vi "S2C_UNITHERM_Proc_Commands.vi"(7 "VI_Ref":refnum<vi>, 8 "Error In":errorcluster, 10 "Settings":T1, 11 "Q-Ref":refnum<queue>) -> (0 "Error Out":errorcluster, 2 "Stop?":bool, 3 "Response":variant)   [LabVIEW 2024]
uses:
  S2C_UNITHERM_Proc_Globals.vi
  _Shared/S2C_Shared_Proc_Globals.vi
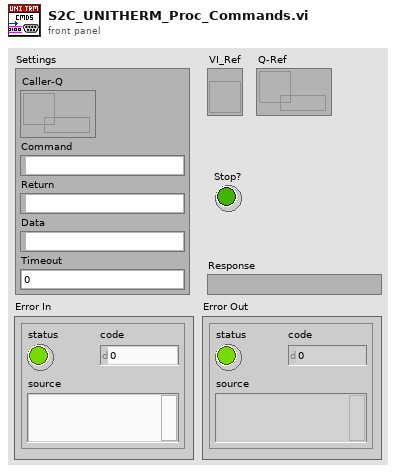
[diagram p1: front panel]
types:
  T1 = cluster{"Caller-Q":refnum<queue>, "Command":string, "Return":string, "Data":variant, "Timeout":dbl}
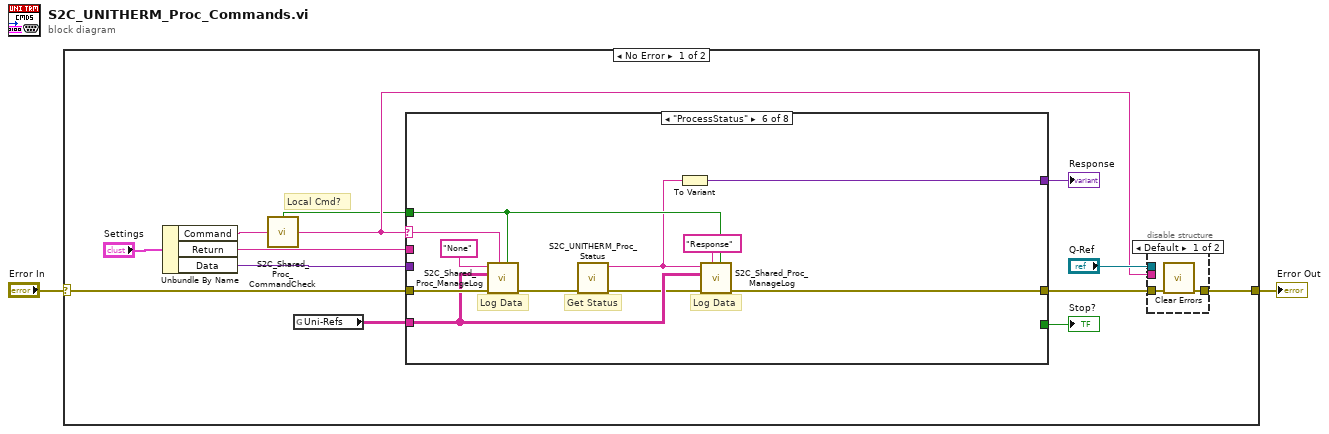
[diagram p0: block diagram]
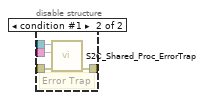
[diagram p2: hidden frame]
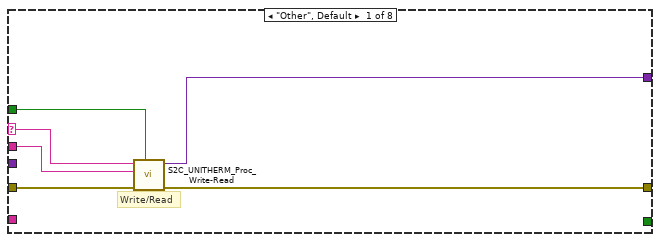
[diagram p3: hidden frame]
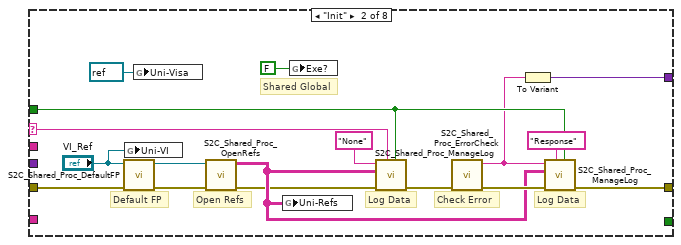
[diagram p4: hidden frame]
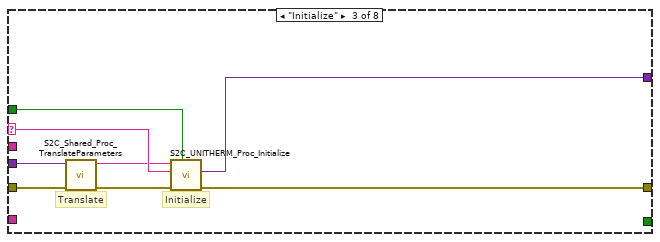
[diagram p5: hidden frame]
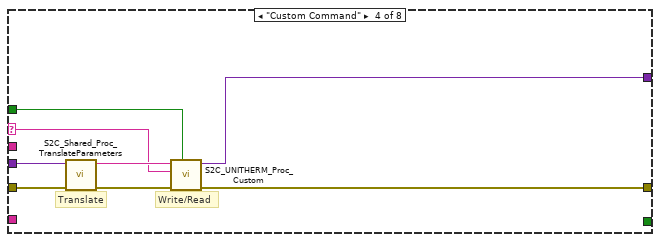
[diagram p6: hidden frame]
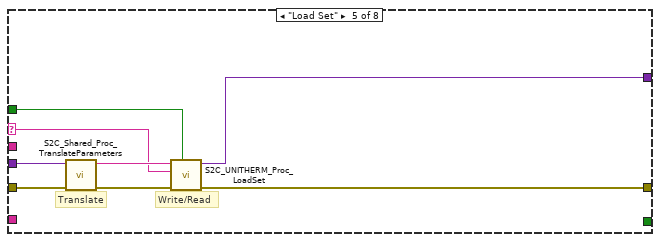
[diagram p7: hidden frame]
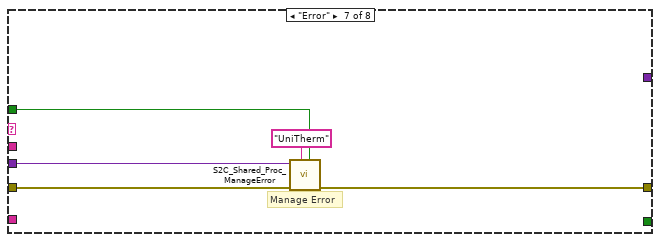
[diagram p8: hidden frame]
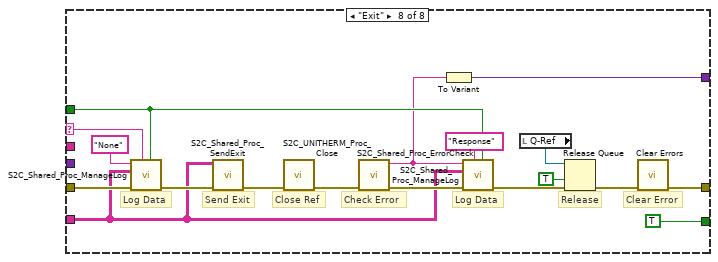
[diagram p9: hidden frame]
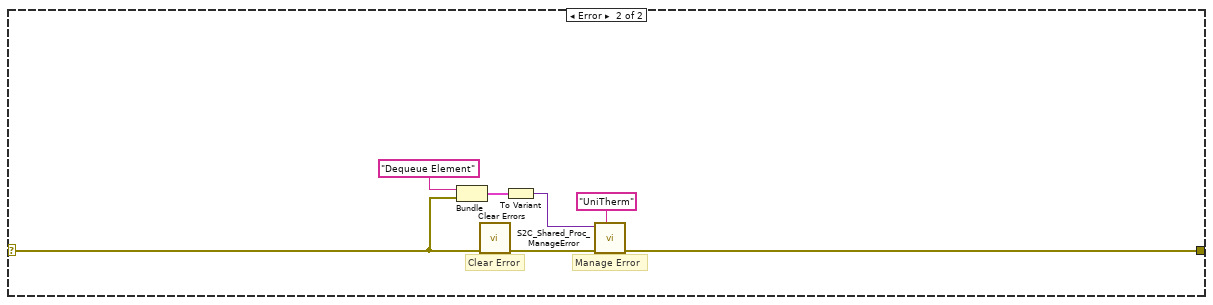
[diagram p10: hidden frame]
diagram:
  n1 = case shown="No Error" "Error In" {
    selector: "Error In" -> [w14 w106]
    tunnel: [w6 w108] -> w1
    frame No Error {
      # "Local Cmd?"
      n2 = Unbundle By Name("Settings") -> ("Command"=w5:string, "Return"=w10:string, "Data"=w15:variant)
      n3 = call "S2C_Shared_Proc_CommandCheck.vi"("Cmd In"=w5) -> ("Local?"=w3:bool, "Cmd Out"=w4:string)  [unwired: 13 in]
      n4 = global read "S2C_UNITHERM_Proc_Globals.vi" "Uni-Refs"() -> (w9:string[][])
      n5 = case shown="\"ProcessStatus\"" w4 {
        selector: w4 -> [w23 w41 w48 w54 w62 w78 _ w99]
        tunnel: w14 -> [w25 w32 w52 w59 w67 w77 w83 w100]
        tunnel: w15 -> [_ _ w51 w58 w66 _ w80 _]
        tunnel: [w27 w44 w50 w60 w68 w74 w82 w85] -> w7
        tunnel: [w26 w38 w49 w57 w65 w75 _ w93] -> w12
        tunnel: [_ _ _ _ _ _ _ TRUE] -> w11
        tunnel: w10 -> [w22 _ _ _ _ _ _ _]
        tunnel: w3 -> [w24 w42 w45 w53 w61 w72 w81 w97]
        tunnel: w9 -> [_ _ _ _ _ w73 _ w90]
        frame "Other", Default {
          # "Write/Read"
          n6 = call "S2C_UNITHERM_Proc_Write-Read.vi"("Local?"=w24, "Error In"=w25, "Return"=w22, "Command"=w23) -> ("Error Out"=w27:errorcluster, "Response"=w26:variant)  [unwired: 6 in]
        }
        frame "Init" {
          # "Default FP"
          # "Shared Global"
          # "Check Error"
          # "Log Data"
          # "Open Refs"
          # "Log Data"
          n7 = call "S2C_Shared_Proc_DefaultFP.vi"("Error In"=w32, "VI_Ref In"="VI_Ref") -> ("Error Out"=w29:errorcluster, "VI_Ref Out"=w30:refnum<vi>)  [unwired: 8 in]
          n8 = global write "S2C_UNITHERM_Proc_Globals.vi" "Uni-VI"("VI_Ref") -> ()
          n9 = global write "S2C_UNITHERM_Proc_Globals.vi" "Uni-Visa"(refnum<visa-resource-name> refnum ("SerialRef")) -> ()
          n10 = call "S2C_Shared_Proc_OpenRefs.vi"("Error In"=w29, "VI_Ref"=w30) -> ("Error Out"=w33:errorcluster, "Refs"=w34:string[][])  [unwired: 8 in]
          n11 = global write "S2C_UNITHERM_Proc_Globals.vi" "Uni-Refs"(w34) -> ()
          n12 = global write "S2C_Shared_Proc_Globals.vi" "Exe?"(FALSE ("Exe?")) -> ()
          n13 = call "S2C_Shared_Proc_ManageLog.vi"("Local?"=w42, "Command"=w41, "Error In"=w33, "Refs"=w34, "Data In"="None") -> ("Error Out"=w36:errorcluster)  [unwired: 5 in, 1 out]
          n14 = call "S2C_Shared_Proc_ErrorCheck.vi"("Error In"=w36) -> ("Error Out"=w39:errorcluster, "Status"=w37:string)  [unwired: 9 in]
          n15 = To Variant(anything=w37) -> (Variant=w38:variant)
          n16 = call "S2C_Shared_Proc_ManageLog.vi"("Local?"=w42, "Command"="Response", "Error In"=w39, "Refs"=w34, "Data In"=w37) -> ("Error Out"=w44:errorcluster)  [unwired: 5 in, 1 out]
        }
        frame "Initialize" {
          # "Initialize"
          # "Translate"
          n17 = call "S2C_Shared_Proc_TranslateParameters.vi"("Error In"=w52, "Data"=w51) -> ("Error Out"=w47:errorcluster, "JSON Cluster"=w46:string)  [unwired: 8 in]
          n18 = call "S2C_UNITHERM_Proc_Initialize.vi"("Local?"=w45, "Error In"=w47, "Command"=w48, "JSON String"=w46) -> ("Error Out"=w50:errorcluster, "Response"=w49:variant)  [unwired: 6 in]
        }
        frame "Custom Command" {
          # "Write/Read"
          # "Translate"
          n19 = call "S2C_Shared_Proc_TranslateParameters.vi"("Error In"=w59, "Data"=w58) -> ("Error Out"=w56:errorcluster, "JSON Cluster"=w55:string)  [unwired: 8 in]
          n20 = call "S2C_UNITHERM_Proc_Custom.vi"("Local?"=w53, "Error In"=w56, "Command"=w54, "JSON String"=w55) -> ("Error Out"=w60:errorcluster, "Response"=w57:variant)  [unwired: 6 in]
        }
        frame "Load Set" {
          # "Write/Read"
          # "Translate"
          n21 = call "S2C_Shared_Proc_TranslateParameters.vi"("Error In"=w67, "Data"=w66) -> ("Error Out"=w64:errorcluster, "JSON Cluster"=w63:string)  [unwired: 8 in]
          n22 = call "S2C_UNITHERM_Proc_LoadSet.vi"("Local?"=w61, "Error In"=w64, "Command"=w62, "JSON String"=w63) -> ("Error Out"=w68:errorcluster, "Response"=w65:variant)  [unwired: 6 in]
        }
        frame "ProcessStatus" {
          # "Get Status"
          # "Log Data"
          # "Log Data"
          n23 = call "S2C_Shared_Proc_ManageLog.vi"("Local?"=w72, "Command"=w78, "Error In"=w77, "Refs"=w73, "Data In"="None") -> ("Error Out"=w71:errorcluster)  [unwired: 5 in, 1 out]
          n24 = call "S2C_UNITHERM_Proc_Status.vi"("Error In"=w71) -> ("Error Out"=w70:errorcluster, "Response"=w69:string)  [unwired: 9 in]
          n25 = To Variant(anything=w69) -> (Variant=w75:variant)
          n26 = call "S2C_Shared_Proc_ManageLog.vi"("Local?"=w72, "Command"="Response", "Error In"=w70, "Refs"=w73, "Data In"=w69) -> ("Error Out"=w74:errorcluster)  [unwired: 5 in, 1 out]
        }
        frame "Error" {
          # "Manage Error"
          n27 = call "S2C_Shared_Proc_ManageError.vi"("Local?"=w81, "Process"="UniTherm", "Error In"=w83, "Data"=w80) -> ("Error Out"=w82:errorcluster)  [unwired: 7 in]
        }
        frame "Exit" {
          # "Clear Error"
          # "Release"
          # "Check Error"
          # "Send Exit"
          # "Log Data"
          # "Close Ref"
          # "Log Data"
          n28 = call "S2C_Shared_Proc_ManageLog.vi"("Local?"=w97, "Command"=w99, "Error In"=w100, "Refs"=w90, "Data In"="None") -> ("Error Out"=w91:errorcluster)  [unwired: 5 in, 1 out]
          n29 = call "S2C_Shared_Proc_SendExit.vi"("Error In"=w91, "Refs"=w90) -> ("Error Out"=w89:errorcluster)  [unwired: 9 in]
          n30 = call "S2C_UNITHERM_Proc_Close.vi"("Error In"=w89) -> ("Error Out"=w98:errorcluster)  [unwired: 10 in]
          n31 = call "S2C_Shared_Proc_ErrorCheck.vi"("Error In"=w98) -> ("Error Out"=w95:errorcluster, "Status"=w92:string)  [unwired: 9 in]
          n32 = To Variant(anything=w92) -> (Variant=w93:variant)
          n33 = call "S2C_Shared_Proc_ManageLog.vi"("Local?"=w97, "Command"="Response", "Error In"=w95, "Refs"=w90, "Data In"=w92) -> ("Error Out"=w94:errorcluster)  [unwired: 5 in, 1 out]
          n34 = local read "Q-Ref"() -> (w87:refnum<queue>)
          n35 = Release Queue(queue=w87, force destroy? (F)=TRUE, error in (no error)=w94) -> (error out=w88:errorcluster)  [unwired: 2 out]
          n36 = call <vilib>:"Clear Errors.vi"("error in (no error)"=w88) -> ("error out"=w85:errorcluster)  [unwired: 5 in, 1 out]
        }
      }
      "Response" <- w12
      "Stop?" <- w11
      n37 = disable-structure shown="Default" {
        disable-tunnel: w7 -> [w17 w21]
        disable-tunnel: [w16 w20] -> w6
        disable-tunnel: w4 -> [_ w19]
        disable-tunnel: "Q-Ref" -> [_ w18]
        frame condition #0 (active) {
          n38 = call <vilib>:"Clear Errors.vi"("error in (no error)"=w17) -> ("error out"=w16:errorcluster)  [unwired: 5 in, 1 out]
        }
        frame condition #1 {
          # "Error Trap"
          n39 = call "S2C_Shared_Proc_ErrorTrap.vi"("Error In"=w21, "Command"=w19, "Q-Ref"=w18) -> ("Error Out"=w20:errorcluster)  [unwired: 8 in]
        }
      }
    }
    frame Error {
      # "Clear Error"
      # "Manage Error"
      n40 = Bundle("Dequeue Element", "error IO"=w106) -> (w107:cluster{string, "error IO":errorcluster})  [unwired: 1 in]
      n41 = call <vilib>:"Clear Errors.vi"("error in (no error)"=w106) -> ("error out"=w103:errorcluster)  [unwired: 5 in, 1 out]
      n42 = To Variant(anything=w107) -> (Variant=w104:variant)
      n43 = call "S2C_Shared_Proc_ManageError.vi"("Process"="UniTherm", "Error In"=w103, "Data"=w104) -> ("Error Out"=w108:errorcluster)  [unwired: 8 in]
    }
  }
  "Error Out" <- w1
